vi "Get Model Path.vi"(3 "Node Path":string) -> (1 "Model Path":string)   [LabVIEW 2016, in "System Mapping Tool.lvlib"]
uses:
  System Mapping Tool.lvlib
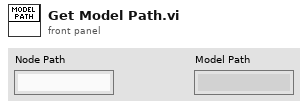
[diagram p1: front panel]
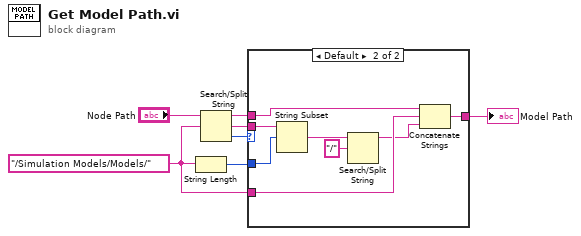
[diagram p0: block diagram]
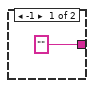
[diagram p2: hidden frame]
diagram:
  w1 = "/Simulation Models/Models/" ("search string/char (-)")
  n1 = String Length(string=w1) -> (length=w5:i32)
  n2 = Search/Split String(string="Node Path", search string/char (-)=w1) -> (substring before match=w2:string, match + rest of string=w6:string, offset of match=w4:i32)  [unwired: 1 in]
  n3 = case shown="Default" w4 {
    tunnel: w6 -> [_ w16]
    tunnel: w5 -> [_ w15]
    tunnel: ["" w9] -> w3
    tunnel: w2 -> [_ w12]
    tunnel: w1 -> [_ w11]
    frame -1 {
    }
    frame Default {
      n4 = String Subset(string=w16, offset (0)=w15) -> (substring=w14:string)  [unwired: 1 in]
      n5 = Search/Split String(string=w14, search string/char (-)="/") -> (substring before match=w10:string)  [unwired: 1 in, 2 out]
      n6 = Concatenate Strings(w12, w11, w10) -> (w9:string)
    }
  }
  "Model Path" <- w3
